vi "DSF.Engine.Memory.Pointer.VS Channels.Write.1D.vi"(7 "count (-1: all)":i64=-1 format="%d elements", 8 "error in (no error)":errorcluster, 9 "offset (0)":u64 format="%d bytes", 10 "Channels Array in":dbl[](array[numeric]), 11 "VS Channels Pointer in":refnum<class "DSF.Engine.Memory.Pointer.VS Channels.lvclass">) -> (0 "error out":errorcluster, 1 "offset out":u64 format="%d bytes", 2 "Channels Array out":dbl[](array[numeric]), 3 "VS Channels Pointer out":refnum<class "DSF.Engine.Memory.Pointer.VS Channels.lvclass">)   [LabVIEW 2016, in "DSF.Engine.lvlib" / "DSF.Engine.Memory.Pointer.VS Channels.lvclass"]
uses:
  DSF.Engine.Memory.Pointer.VS Channels.lvclass
  C:/Git/Sourcetree/DSF/Source/Submodules/Memory Manager/Source/Classes/Pointer/Memory.Pointer.lvclass
  DSF.Engine.Memory.Pointer.VS Channels.lvclass/DSF.Engine.Memory.Pointer.VS Channels.ctl
  Submodules/Memory Manager/Source/Classes/Pointer/Memory.Pointer.lvclass/Memory.Pointer.ctl
  Submodules/Memory Manager/Source/Classes/Pointer/Methods/Memory.Pointer.Write.Safe.1D.DBL.vi
  Submodules/Memory Manager/Source/Classes/Pointer/Methods/Memory.Pointer.Write.Unsafe.1D.DBL.vi
  Submodules/Memory Manager/Source/Classes/Pointer/Methods/Memory.Pointer.Parameter Check.Null Pointer.vi
  Submodules/Memory Manager/Source/Classes/Pointer/Methods/Memory.Pointer.Parameter Check.Subset.Power of 2.vi
  Submodules/Memory Manager/Source/Classes/Pointer/Accessors/Get Address.vi
  Submodules/Memory Manager/Source/Classes/Pointer/Methods/Memory.Pointer.Errors.vi
  Submodules/Memory Manager/Source/Classes/Pointer/Methods/Memory.Pointer.Errors.Null Pointer.vi
  Submodules/Memory Manager/Source/Classes/Pointer/Methods/Memory.Pointer.Errors.Out of Bounds.vi
  Submodules/Memory Manager/Source/Classes/Pointer/Accessors/Get Size.vi
  Submodules/Memory Manager/Source/VIs/Memory.Count to Size.Power of 2.vi
  Submodules/Memory Manager/Source/Classes/Pointer/Methods/Memory.Pointer.Errors.Create Error.vi
  Submodules/Memory Manager/Source/Submodules/SEH/Source/VIs/Static Error Handling.Source Buffer.Write.String.vi
  Submodules/Memory Manager/Source/Classes/Pointer/Methods/Memory.Pointer.Errors.Write Pointer Size.vi
  Submodules/Memory Manager/Source/Submodules/SEH/Source/VIs/Static Error Handling.Source Buffer.Write.Numeric.Scalar.Base10.vi
  Submodules/Memory Manager/Source/Submodules/SEH/Source/VIs/Static Error Handling.Source Buffer.Write.Numeric.Scalar.Base10 (U64).vi
  Submodules/Memory Manager/Source/Submodules/SEH/Source/VIs/Static Error Handling.Error Cluster Constant.vi
  Submodules/Memory Manager/Source/Submodules/SEH/Source/VIs/Static Error Handling.Error Cluster Constant (256B).vi
  Submodules/Memory Manager/Source/Submodules/SEH/Source/VIs/Static Error Handling.Parameters.Status.Set.vi
  Submodules/Memory Manager/Source/Submodules/SEH/Source/VIs/Static Error Handling.Parameters.Code.Set.vi
  Submodules/Memory Manager/Source/Submodules/SEH/Source/VIs/Static Error Handling.Parameters.VI Source.Set.vi
  Submodules/Memory Manager/Source/Constants/Memory.Constants.vi
  Submodules/Memory Manager/Source/Constants/Memory.Constants.Library Name.vi
  Submodules/Memory Manager/Source/Classes/Pointer/Methods/Memory.Pointer.Errors.Get Info.vi
  Submodules/Memory Manager/Source/Classes/Pointer/Memory.Pointer.lvclass
  C:/Git/Sourcetree/DSF/Source/Submodules/Memory Manager/Source/Classes/Pointer.External/Memory.Pointer.External.lvclass
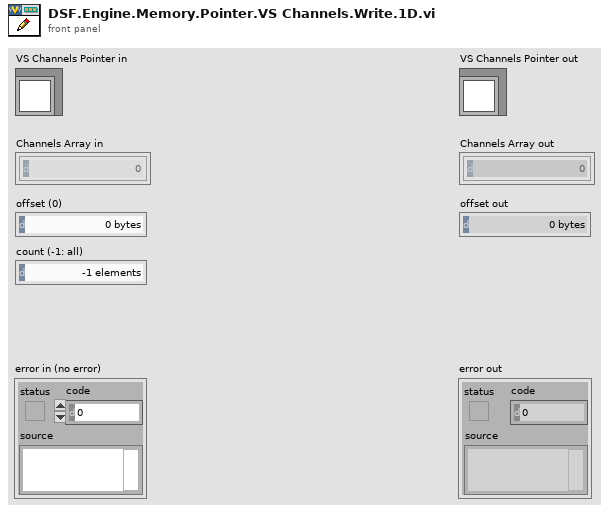
[diagram p1: front panel]
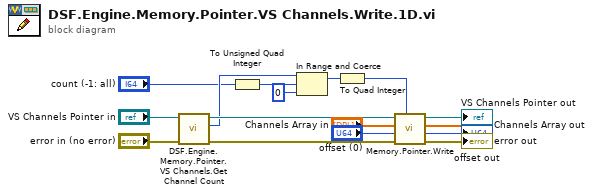
[diagram p0: block diagram]
diagram:
  n1 = call "DSF.Engine.Memory.Pointer.VS Channels.Get Channel Count.vi"("error in (no error)"="error in (no error)", "VS Channels Pointer in"="VS Channels Pointer in") -> ("error out"=w16:errorcluster, "channel count"=w7:u64, "VS Channels Pointer out"=w13:refnum<class "DSF.Engine.Memory.Pointer.VS Channels.lvclass">)  [unwired: 7 in]
  n2 = To Unsigned Quad Integer(1:"count (-1: all)") -> (0:w5:u64)
  n3 = In Range and Coerce(upper limit=w7, x=w5, lower limit=u64 0) -> (coerced(x)=w3:u64)  [unwired: 1 out]
  n4 = To Quad Integer(1:w3) -> (0:w2:i64)
  n5 = call-poly "Memory.Pointer.Write.vi"("count (-1: all)"=w2, "error in (no error)"=w16, "offset (0)"="offset (0)", "buffer in"="Channels Array in", "pointer in"=w13) -> ("error out"=→"error out":errorcluster, "offset out"=→"offset out":u64, "buffer out"=→"Channels Array out":dbl[], "pointer out"=→"VS Channels Pointer out":refnum<class "DSF.Engine.Memory.Pointer.VS Channels.lvclass">)  [unwired: 3 in]
